vi "状态机-骰子-1.vi"() -> ()   [LabVIEW 2023]
uses:
  <vilib>/numeric/Random Number (Range) U64.vi
  <vilib>/numeric/sub_Random U32.vi
panel:
  in  "print":bool
  out "Waveform Chart":u64(graph)
  in  "stop":bool
  in  "Throw Dice":bool
  out "Numeric":u64
  # "状态记 骰子"
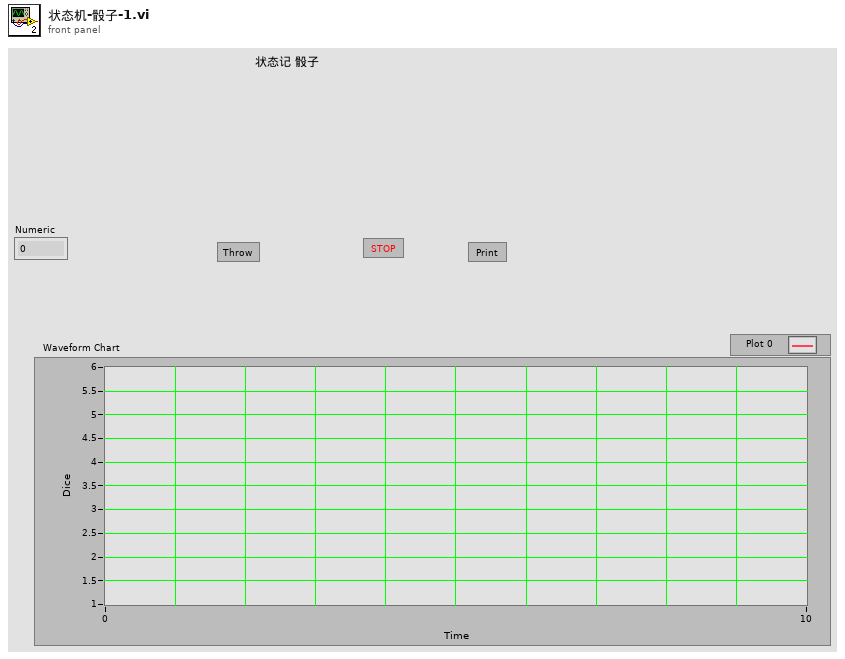
[diagram p1: front panel]
types:
  T1 = typedef "imagedata.ctl" = cluster{"image type":i32, "image depth":i32, "image":u8[], "mask":u8[], "colors":u32[], "Rectangle":cluster{"left":i16, "top":i16, "right":i16, "bottom":i16}}
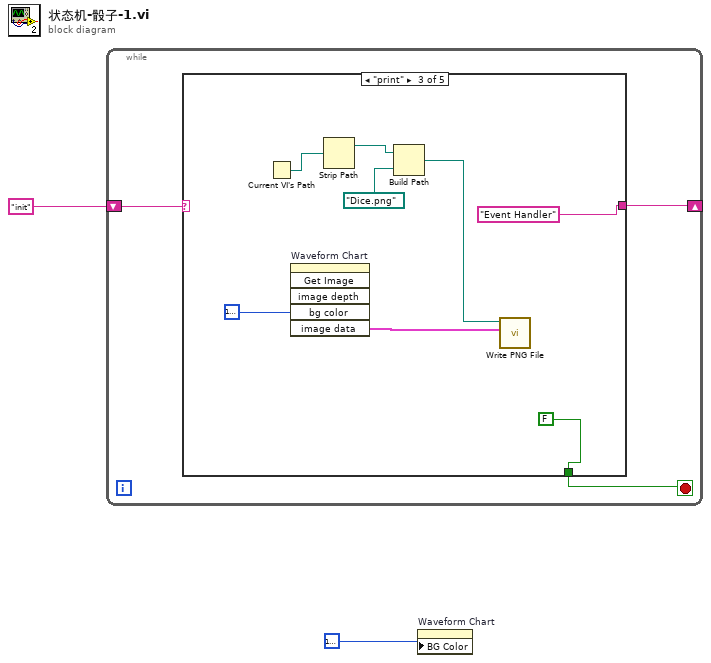
[diagram p0: block diagram]
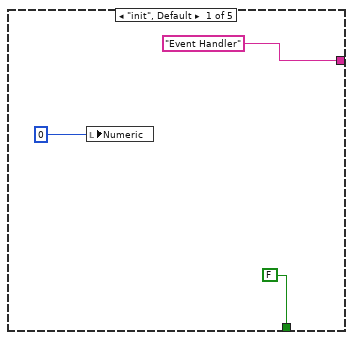
[diagram p2: hidden frame]
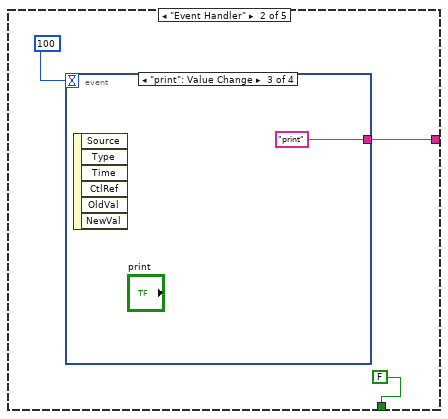
[diagram p3: hidden frame]
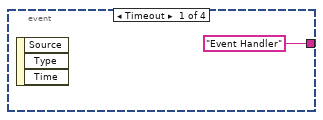
[diagram p4: hidden frame]
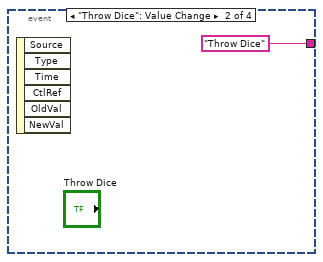
[diagram p5: hidden frame]
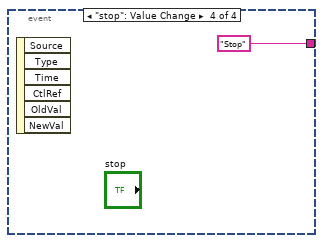
[diagram p6: hidden frame]
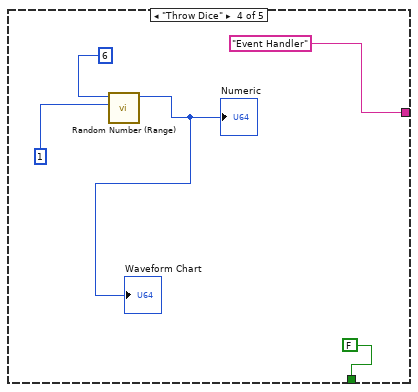
[diagram p7: hidden frame]
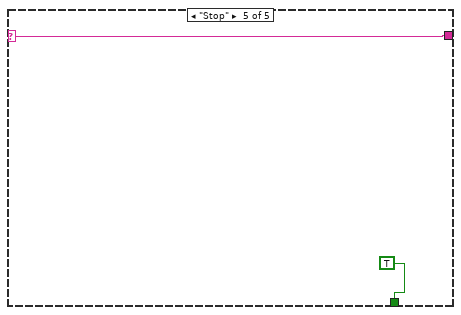
[diagram p8: hidden frame]
diagram:
  n1 = while {
    shift-right: [w4] -> _
    shift-left: "init" -> [w5]
    stop <- w3 stop-if-true
    n2 = case shown="\"print\"" w5 {
      selector: w5 -> [_ _ _ _ w30]
      tunnel: ["Event Handler" w10 "Event Handler" "Event Handler" w30] -> w4
      tunnel: [FALSE FALSE FALSE FALSE TRUE] -> w3
      frame "init", Default {
        n3 = local write "Numeric"(u64 0 ("Numeric")) -> ()
      }
      frame "Event Handler" {
        n4 = event shown="[2] \"print\": Value Change" {
          selector: _ -> [_ _ _ _]
          dyn-events: _ -> [_ _ _ _]
          timeout: 100 -> [_ _ _ _]
          tunnel: ["Event Handler" "Throw Dice" "print" "Stop"] -> w10
          event Timeout {
            n5 = event-data() -> ()  [unwired: 1 in, 3 out]
          }
          event "Throw Dice": Value Change {
            n6 = event-data() -> ()  [unwired: 1 in, 6 out]
          }
          event "print": Value Change {
            n7 = event-data() -> ()  [unwired: 1 in, 6 out]
          }
          event "stop": Value Change {
            n8 = event-data() -> ()  [unwired: 1 in, 6 out]
          }
        }
      }
      frame "print" {
        n9 = Current VI's Path() -> (path=w19:path)
        n10 = invoke on="Waveform Chart" class="WFChart (strict)" method="Get Image"("bg color"=u32 16777238) -> ("image data"=w20:T1)  [unwired: 5 in, 5 out]
        n11 = Strip Path(path=w19) -> (stripped path=w18:path)  [unwired: 1 out]
        n12 = Build Path(base path=w18, name or relative path=path "Dice.png") -> (appended path=w16:path)
        n13 = call <vilib>:"Write PNG File.vi"("image data"=w20, "path to PNG file"=w16) -> ()  [unwired: 8 in, 2 out]
      }
      frame "Throw Dice" {
        n14 = call-poly <vilib>:"Random Number (Range).vi"("lower bound (0)"=u64 1, "upper bound (100)"=u64 6) -> ("number"=→"Numeric" →"Waveform Chart":u64)  [unwired: 9 in]
      }
      frame "Stop" {
      }
    }
  }
  n15 = property on="Waveform Chart" class="WFChart (strict)"("BG Color"=u32 16777238) -> ()  [unwired: 2 in, 2 out]
